vi "Install.vi"   [LabVIEW 2015]
uses:
  FPGAChannelsManager/FPGAChannelsManager.lvclass
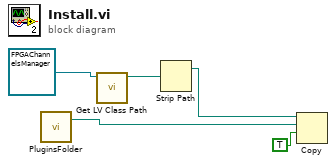
[diagram p0: block diagram]
diagram:
  n1 = call <resource>:"PluginsFolder.vi"() -> ("PluginsFolderPath"=w1:path)  [unwired: 3 in]
  n2 = call <vilib>:"Get LV Class Path.vi"("object"=refnum<class "FPGAChannelsManager.lvclass"> refnum ("ClassMethodsInheritance")) -> ("class path"=w4:path)  [unwired: 9 in, 1 out]
  n3 = Strip Path(path=w4) -> (stripped path=w3:path)  [unwired: 1 out]
  n4 = Copy(9:TRUE ("overwrite (F)"), 10:w1, 11:w3) -> ()  [unwired: 2 in, 3 out]
